vi "IsHotGoal.vi"(8 "error in":errorcluster, 9 "% Cutoff":dbl, 10 "Num samples":i32) -> (0 "error out":errorcluster, 2 "Hot/Not":bool)   [LabVIEW 2013]
doc: "IsHotGoal checks if the goal is hot at the beginning of autonomous mode.\n-NumSamples determines how many images of the goal the camera will process.\n-% Cutoff (meant to be a decimal value) determines the minimum ratio of hot images/total images needed for IsHotGoal to report a hot goal."
uses:
  Example_Code/2014 Target Detection/TargetType.ctl
panel:
  in  "Color System":u16(ring)=2 items=["RGB", "HSL", "HSV", "HSI"]
  in  "Score cutoff":dbl=50.0
  out "Distance (ft)":dbl
  out "Scores.State":T1
  in  "Color Components":T2={"Hue"={116.0, 148.0}, "Sat"={152.0, 255.0}, "Val"={237.0, 255.0}} {"Val" scale=0.0..255.0; "Sat" scale=0.0..255.0; "Hue" scale=0.0..255.0 scale format="%#_3g"}
  out "Time (ms)":u32
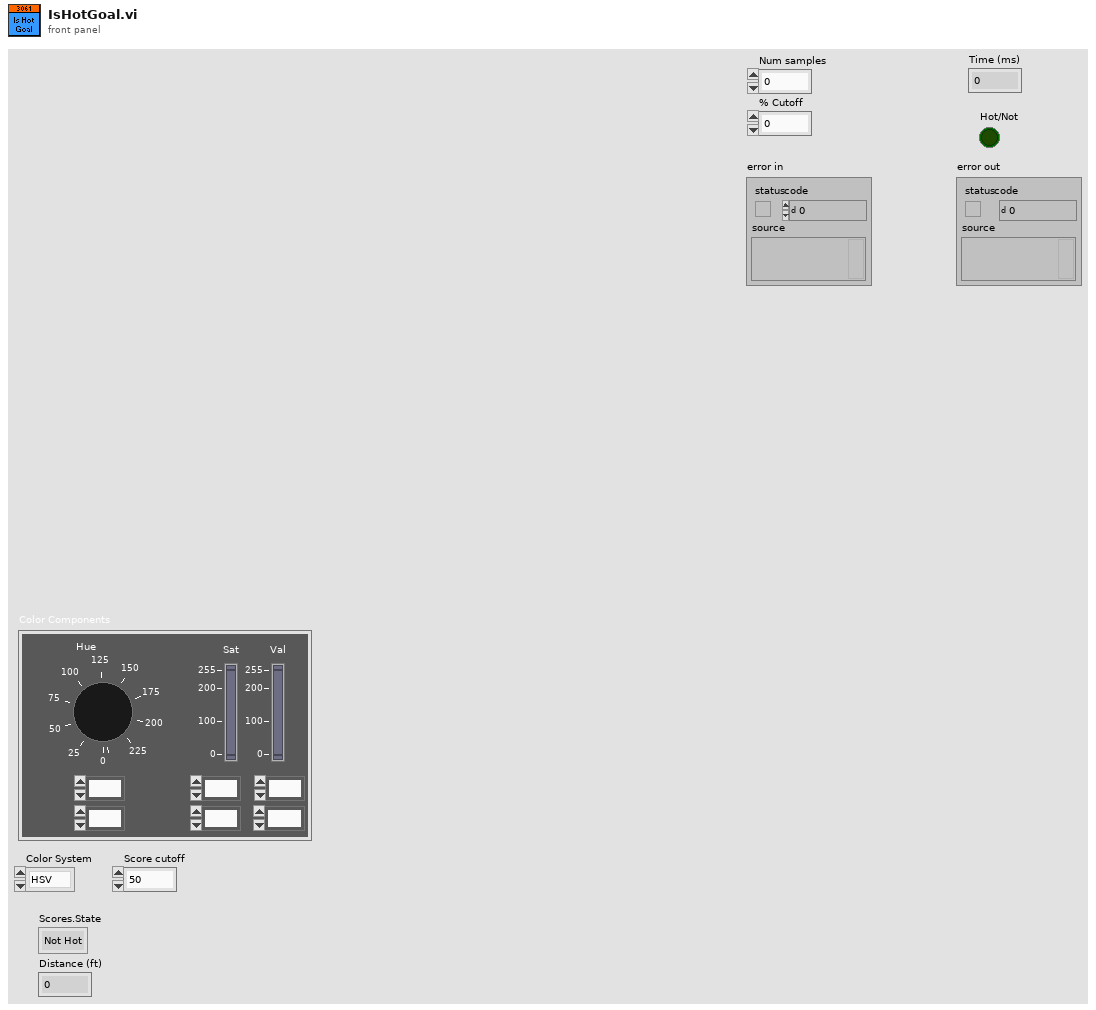
[diagram p1: front panel]
types:
  T1 = typedef "TargetType.ctl" = enum16{"Not Hot", "Hot"}
  T2 = cluster{"Hue":cluster{dbl, dbl}, "Sat":cluster{dbl, dbl}, "Val":cluster{dbl, dbl}}
  T3 = typedef "Image Type" = u32
  T4 = typedef "WPI_CameraDevRef.ctl" = cluster{"Camera Address":string, "CameraStatus":errorcluster, "Acquire Image Notifier":refnum<notifier>}
  T5 = typedef "IMAQ Image.ctl" = refnum<image>
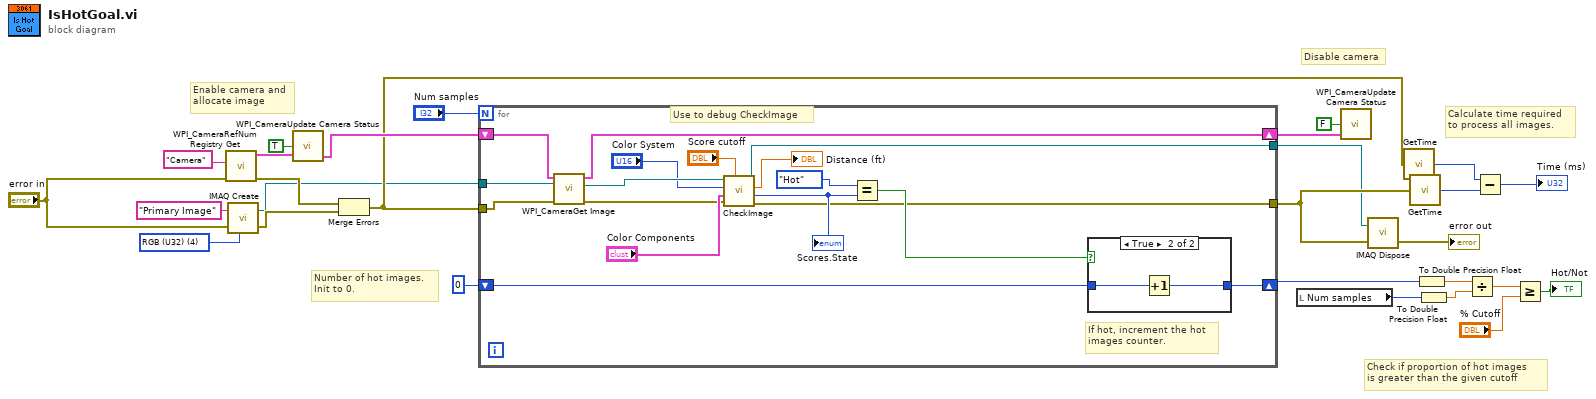
[diagram p0: block diagram]
diagram:
  w12 = T3 4 items=["Grayscale (U8)", "Grayscale (I16)", "Grayscale (SGL)", "Complex (CSG)", "RGB (U32)", "HSL (U32)", "RGB (U64)"] ("Image Type")
  # "Disable camera"
  # "Enable camera and\nallocate image"
  # "Calculate time required \nto process all images."
  # "Check if proportion of hot images\nis greater than the given cutoff"
  # "Number of hot images.\nInit to 0."
  n1 = call <vilib>:"WPI_CameraRefNum Registry Get.vi"("error in (no error)"="error in", "refnum name"="Camera") -> ("error out"=w8:errorcluster, "CameraDevRef"=w15:T4)  [unwired: 8 in]
  n2 = call "IMAQ Create"("Image Name"="Primary Image", "Image Type"=w12, "error in (no error)"="error in") -> ("New Image"=w6:T5, "error out"=w9:errorcluster)  [unwired: 1 in, 1 out]
  n3 = call <vilib>:"WPI_CameraUpdate Camera Status.vi"("CameraDevRef In"=w15, "Enable Vision"=TRUE) -> ("CameraDevRef Out"=w13:T4)  [unwired: 3 in]
  n4 = Merge Errors(w8, w9) -> (w7:errorcluster)
  n5 = for {
    N: "Num samples" -> [_]
    tunnel: w7 -> [w34]
    shift-right: [w44] -> w23
    shift-left: 0 ("Num samples 2") -> [w45]
    tunnel: [w31] -> w3
    tunnel: w6 -> [w35]
    shift-right: [w30] -> w5
    shift-left: w13 -> [w33]
    tunnel: [w29] -> w1
    # "Use to debug CheckImage"
    # "If hot, increment the hot\nimages counter."
    n6 = call <vilib>:"WPI_CameraGet Image.vi"("error in (no error)"=w34, "Image"=w35, "CameraDevRef"=w33) -> ("error out"=w32:errorcluster, "Image Out"=w43:T5, "CameraDevRef Out"=w30:T4)  [unwired: 6 out]
    n7 = call "CheckImage.vi"("Score cutoff"="Score cutoff", "error in"=w32, "Color Components"="Color Components", "Color System"="Color System", "Image"=w43) -> ("error out"=w31:errorcluster, "Scores.State"=w37:T1, "Distance (ft)"=→"Distance (ft)":dbl, "Image out"=w29:T5)  [unwired: 3 in]
    "Scores.State" <- w37
    n8 = Equal?(x=TargetType."Hot" ("Scores.State 2"), y=w37) -> (x = y?=w36:bool)
    n9 = case shown="True" w36 {
      tunnel: w45 -> [w46 w48]
      tunnel: [w46 w47] -> w44
      frame False {
      }
      frame True {
        n10 = Increment(x=w48) -> (x+1=w47:i32)
      }
    }
  }
  n11 = local read "Num samples"() -> (w22:i32)
  n12 = call <vilib>:"WPI_CameraUpdate Camera Status.vi"("CameraDevRef In"=w5, "Enable Vision"=FALSE) -> ()  [unwired: 3 in, 1 out]
  n13 = call "IMAQ Dispose"("Image"=w1, "error in (no error)"=w3) -> ("error out"=→"error out":errorcluster)  [unwired: 4 in]
  n14 = call "GetTime.vi"("error in"=w7) -> ("Time"=w17:u32)
  n15 = call "GetTime.vi"("error in"=w3) -> ("Time"=w18:u32)
  n16 = To Double Precision Float(number=w23) -> (double precision float=w20:dbl)
  n17 = To Double Precision Float(number=w22) -> (double precision float=w21:dbl)
  n18 = Divide(x=w20, y=w21) -> (x/y=w24:dbl)
  n19 = Subtract(x=w17, y=w18) -> (x-y=→"Time (ms)":u32)
  n20 = Greater Or Equal?(x=w24, y="% Cutoff") -> (x >= y?=→"Hot/Not":bool)
